vi "spi_trial.vi"() -> ()   [LabVIEW 2024]
uses:
  <vilib>/MakerHub/LINX/Private/Type Defs/Peripherals/SPI/SPI Configuration.ctl
  <vilib>/MakerHub/LINX/Private/Type Defs/Peripherals/SPI/SPI Bit Order.ctl
  <vilib>/MakerHub/LINX/Private/Type Defs/Peripherals/SPI/SPI Mode.ctl
  <vilib>/MakerHub/LINX/Public/Peripherals/SPI/SPI CS Config.ctl
  <vilib>/MakerHub/LINX/Private/Type Defs/Peripherals/SPI/SPI CS Logic Level.ctl
  <vilib>/MakerHub/LINX/Private/Local IO/LinxSpiWriteRead.vi
  <vilib>/MakerHub/LINX/Public/Utilities/Check Channel.vi
  <vilib>/MakerHub/LINX/Public/Utilities/Open Serial.vi
  <vilib>/MakerHub/LINX/Private/Utilties/Generate Error.vi
  <vilib>/MakerHub/LINX/LMH-LINX.lvlib
  <vilib>/MakerHub/LINX/Public/Peripherals/SPI/SPI Write Read 1 Frame.vi
panel:
  out "Error Out":errorcluster
  out "Read Data":u8[](array[numeric])
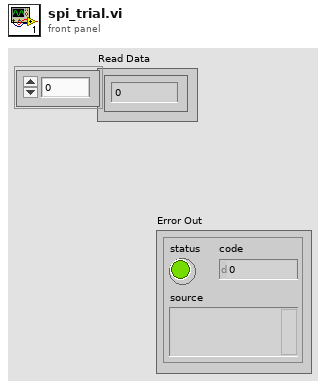
[diagram p1: front panel]
types:
  T1 = typedef "LMH-LINX.lvlib/SPI CS Config.ctl" = cluster{"CS Channel":u8, "CS Logic Level":T2}
  T2 = typedef "LMH-LINX.lvlib/SPI CS Logic Level.ctl" = enum8{"Active Low", "Active High"}
  T3 = typedef "LMH-LINX.lvlib/SPI Configuration.ctl" = cluster{"Clock Frequency":u32, "Bit Order":T4, "SPI Mode":T5}
  T4 = typedef "LMH-LINX.lvlib/SPI Bit Order.ctl" = enum8{"LSb First", "MSb First"}
  T5 = typedef "LMH-LINX.lvlib/SPI Mode.ctl" = enum8{"Mode 0", "Mode 1", "Mode 2", "Mode 3"}
  T6 = typedef "LMH-LINX.lvlib/LINX Ref.ctl" = cluster{"IO":T7, "Interface":T8, "LINX Device Config":T9}
  T7 = typedef "LMH-LINX.lvlib/Platform.ctl" = enum16{"Remote", "Local"}
  T8 = typedef "LMH-LINX.lvlib/Interface.ctl" = enum16{"Serial", "TCP"}
  T9 = typedef "LMH-LINX.lvlib/Device.lvlib/LINX Device Config.ctl" = cluster{"Interface":T8, "COM Port":refnum<visa-resource-name>, "TCP Configuration":T10, "Device Family":u8, "Device ID":u8, "Device Name":string, "TCP Ref":refnum<k5>, "Channels":T11}
  T10 = typedef "LMH-LINX.lvlib/Device.lvlib/TCP Config.ctl" = cluster{"IP Address":string, "Port":u16}
  T11 = typedef "LMH-LINX.lvlib/Channels.ctl" = cluster{"DI":u8[], "DO":u8[], "AI":u8[], "AO":u8[], "PWM":u8[], "QE":u8[], "UART":u8[], "I2C 2":u8[], "SPI":u8[], "CAN":u8[], "Servo":u8[], "AI Ref (V)":dbl, "AI Resolution (Bits)":u8, "AO Ref (V)":dbl, "AO Resolution (Bits)":u8}
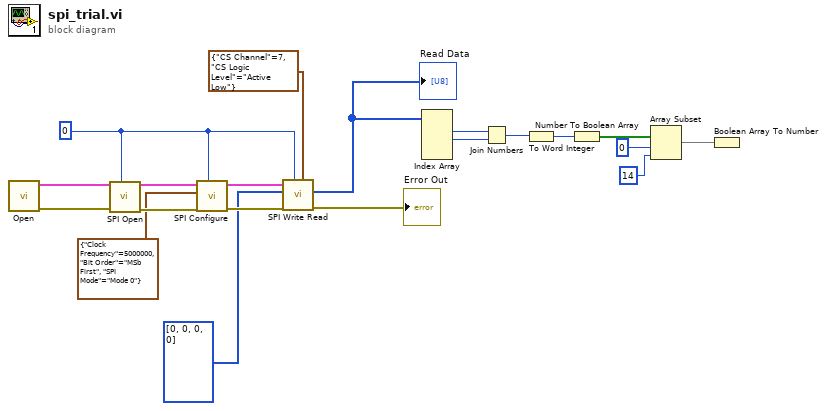
[diagram p0: block diagram]
diagram:
  w4 = 0
  n1 = call-poly <vilib>:"Open.vi"() -> ("Error Out"=w19:errorcluster, "LINX Resource"=w20:T6)  [unwired: 9 in, 1 out]
  n2 = call <vilib>:"SPI Open.vi"("SPI Channel (0)"=w4, "Error In"=w19, "LINX Resource"=w20) -> ("Error Out"=w18:errorcluster, "LINX Resource"=w17:T6)  [unwired: 7 in]
  n3 = call <vilib>:"SPI Configure.vi"("SPI Channel (0)"=w4, "Error In"=w18, "SPI Configuration"=T3 {"Clock Frequency"=5000000, "Bit Order"=enum."MSb First", "SPI Mode"=enum."Mode 0"}, "LINX Resource"=w17) -> ("Error Out"=w16:errorcluster, "LINX Resource"=w15:T6)  [unwired: 5 in, 1 out]
  n4 = call-poly <vilib>:"SPI Write Read.vi"("CS Configuration"=T1 {"CS Channel"=7, "CS Logic Level"=enum."Active Low"}, "SPI Channel (0)"=w4, "Error In"=w16, "Data"=u8[] [0, 0, 0, 0], "LINX Resource"=w15) -> ("Error Out"=→"Error Out":errorcluster, "Read Data"=w13:u8[])  [unwired: 3 in, 2 out]
  "Read Data" <- w13
  n5 = Index Array(array=w13) -> (element #1=w11:u8, element #2=w10:u8)  [unwired: 4 in, 2 out]
  n6 = Join Numbers(hi=w11, lo=w10) -> ((hi.lo)=w9:u16)
  n7 = To Word Integer(number=w9) -> (16bit integer=w8:i16)
  n8 = Number To Boolean Array(number=w8) -> (Boolean array=w7:bool[])
  n9 = Array Subset(array=w7, index=0, length=14) -> (w1:bool[])
  n10 = Boolean Array To Number(Boolean array=w1) -> ()  [unwired: 1 out]
